vi "libssh2_scp_recv2.vi"(8 "error in (no error)":errorcluster, 10 "path":string, 11 "session":T3) -> (0 "error out":errorcluster, 2 "stat":T1, 3 "channel":T2)   [LabVIEW 2013, in "libssh2.lvlib"]
doc: "Request a file from an SSH server. When successful, returns a channel instance and the remote file's size, mode, mtime, and atime."
uses:
  libssh2.lvlib
  Session Refnum.ctl
  Channel Refnum.ctl
  libssh2_struct_stat.ctl
  Not A Session.vi
  <vilib>/Utility/error.llb/Error Cluster From Error Code.vi
  Global Settings.vi
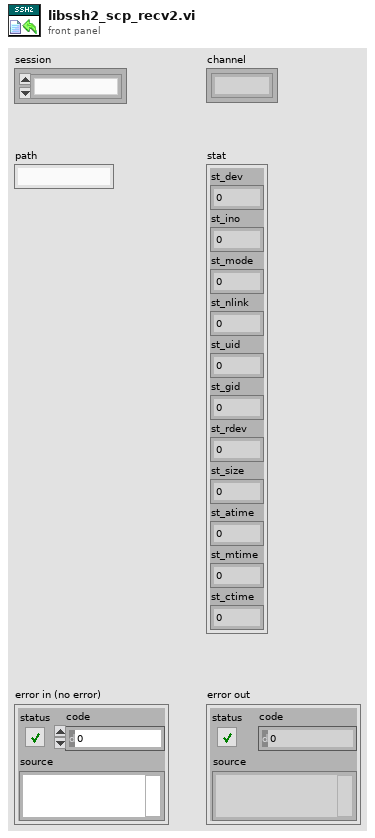
[diagram p1: front panel]
types:
  T1 = typedef "libssh2.lvlib/libssh2_struct_stat.ctl" = cluster{"st_dev":u64, "st_ino":u16, "st_mode":u16, "st_nlink":i16, "st_uid":i16, "st_gid":i16, "st_rdev":u32, "st_size":i64, "st_atime":i64, "st_mtime":i64, "st_ctime":i64}
  T2 = typedef "libssh2.lvlib/Channel Refnum.ctl" = refnum<k1>
  T3 = typedef "libssh2.lvlib/Session Refnum.ctl" = refnum<k1>
  T4 = cluster{"st_dev":u64, "st_ino":u16, "st_mode":u16, "st_nlink":i16, "st_uid":i16, "st_gid":i16, "<padding>":i16, "st_rdev":u32, "st_size":i64, "st_atime":i64, "st_mtime":i64, "st_ctime":i64}
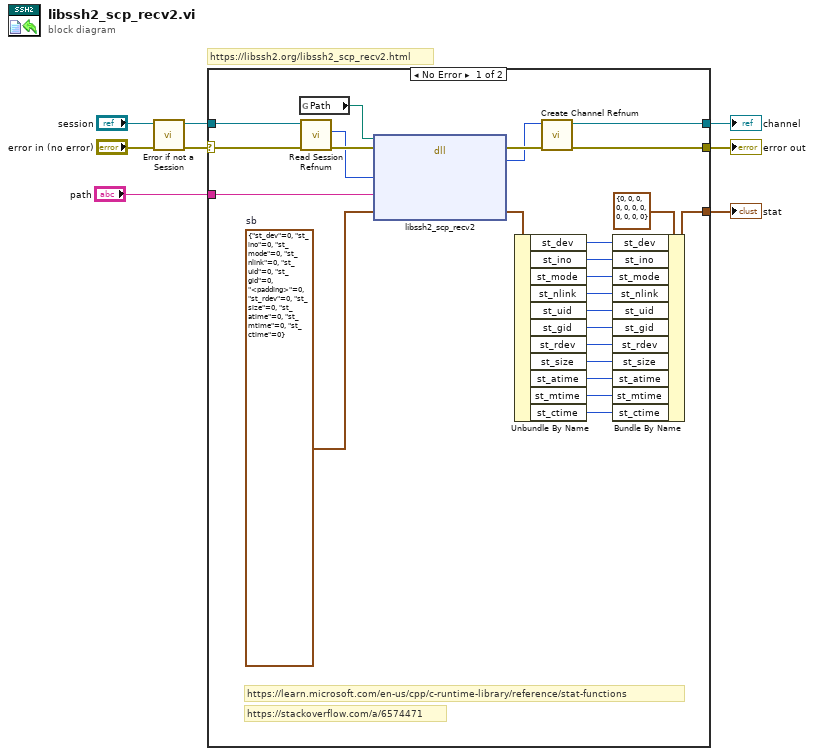
[diagram p0: block diagram]
diagram:
  # "https://libssh2.org/libssh2_scp_recv2.html"
  n1 = call "Error if not a Session.vi"("error in (no error)"="error in (no error)", "session"="session") -> ("error out"=w5:errorcluster, "session out"=w3:T3)  [unwired: 8 in]
  n2 = case shown="No Error" w5 {
    selector: w5 -> [w26 w34]
    tunnel: w3 -> [w31 _]
    tunnel: [w29 w34] -> w8
    tunnel: [w27 _] -> w7
    tunnel: "path" -> [w24 _]
    tunnel: [w9 _] -> w1
    frame No Error {
      w23 = T4 {"st_dev"=0, "st_ino"=0, "st_mode"=0, "st_nlink"=0, "st_uid"=0, "st_gid"=0, "<padding>"=0, "st_rdev"=0, "st_size"=0, "st_atime"=0, "st_mtime"=0, "st_ctime"=0}  # sb
      # "https://stackoverflow.com/a/6574471"
      # "https://learn.microsoft.com/en-us/cpp/c-runtime-library/reference/stat-functions"
      n3 = global read "Global Settings.vi" "Path"() -> (w25:path)
      n4 = call "Read Session Refnum.vi"("error in (no error)"=w26, "session"=w31) -> ("error out"=w32:errorcluster, "LIBSSH2_SESSION*"=w30:u64)  [unwired: 5 in, 3 out]
      n5 = dll-call lib="?" fn="libssh2_scp_recv2"(path in=w25, error in=w32, "session"=w30, "path"=w24, "sb"=w23) -> (error out=w33:errorcluster, "return value"=w28:u64, "sb"=w22:T4)  [unwired: 3 in, 1 out]
      n6 = Unbundle By Name(w22) -> ("st_dev"=w20:u64, "st_ino"=w19:u16, "st_mode"=w18:u16, "st_nlink"=w17:i16, "st_uid"=w16:i16, "st_gid"=w15:i16, "st_rdev"=w14:u32, "st_size"=w13:i64, "st_atime"=w12:i64, "st_mtime"=w11:i64, "st_ctime"=w10:i64)
      n7 = call "Create Channel Refnum.vi"("error in (no error)"=w33, "LIBSSH2_CHANNEL*"=w28) -> ("error out"=w29:errorcluster, "channel"=w27:T2)  [unwired: 8 in]
      n8 = Bundle By Name(cluster=T1 {"st_dev"=0, "st_ino"=0, "st_mode"=0, "st_nlink"=0, "st_uid"=0, "st_gid"=0, "st_rdev"=0, "st_size"=0, "st_atime"=0, "st_mtime"=0, "st_ctime"=0} ("sb"), "st_dev"=w20, "st_ino"=w19, "st_mode"=w18, "st_nlink"=w17, "st_uid"=w16, "st_gid"=w15, "st_rdev"=w14, "st_size"=w13, "st_atime"=w12, "st_mtime"=w11, "st_ctime"=w10) -> (w9:T1)
    }
    frame Error {
    }
  }
  "error out" <- w8
  "channel" <- w7
  "stat" <- w1
